vi "setTemperatureSetpoint.vi"(8 "error in (no error)":errorcluster, 10 "Device":i32, 11 "SEDSpectrometer in":refnum<class "FiberSpectrograph.lvclass">) -> (0 "error out":errorcluster, 3 "SEDSpectrometer out":refnum<class "FiberSpectrograph.lvclass">)   [LabVIEW 2016, in "FiberSpectrograph.lvclass"]
uses:
  FiberSpectrograph.lvclass
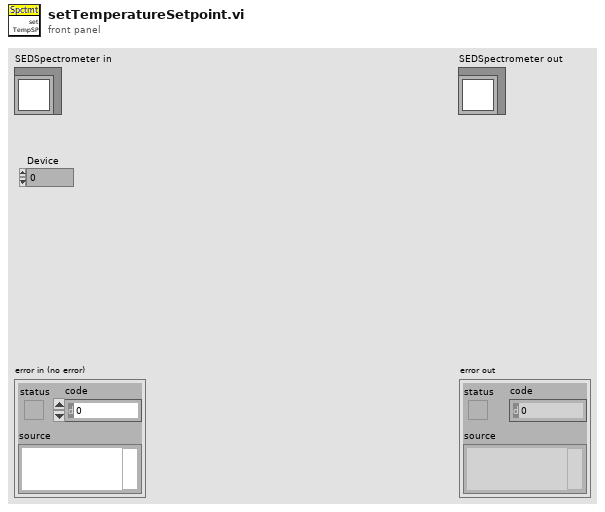
[diagram p1: front panel]
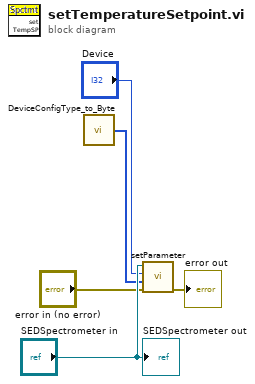
[diagram p0: block diagram]
diagram:
  n1 = call "DeviceConfigType_to_Byte.vi"() -> ("Byte Array"=w4:u8[])  [unwired: 5 in]
  n2 = call "setParameter.vi"("error in (no error)"="error in (no error)", "DeviceParm"=w4, "Device"="Device", "SEDSpectrometer in"="SEDSpectrometer in") -> ("error out"=→"error out":errorcluster)  [unwired: 4 in, 3 out]
  "SEDSpectrometer out" <- "SEDSpectrometer in"
